vi "LSRS Drive.vi"(7 "Drive Side":enum16{"Right Side", "Left Side "}(ring), 10 "Inputs":dbl[](array[numeric])) -> (1 "Current Speed":dbl, 2 "Motor 2 Output":dbl, 3 "Motor Output":dbl)   [LabVIEW 2016]
uses:
  <vilib>/Rock Robotics/Network Tables/NT Read Number.vi
  <vilib>/Rock Robotics/Network Tables/NT Write Number.vi
  <vilib>/addons/control/pid/pid.llb/PID (DBL).vi
  <vilib>/addons/control/pid/NI_PID_pid.lvlib
panel:
  out "PID Values":cluster{"P":dbl, "I":dbl, "D":dbl}
  out "Right Button":bool
  out "Left Button":bool
  # "Left/Right Side Drive \nFRC Team 6364"
  # "Red is left side on."
  # "Blue is right side on."
  # "Adapted from Team 34`s Program"
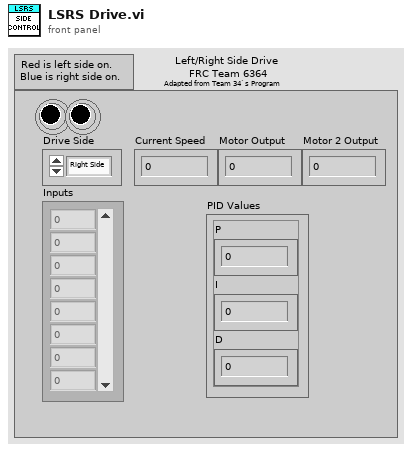
[diagram p1: front panel]
types:
  T1 = enum16{"Z", "Y", "X", "Rot. Point X", "Rot. Point Y", "Width/2", "Max", "Length/2"}
  T2 = typedef "WPI_EncoderDevRef.ctl" = cluster{"DevStatus":errorcluster, "EncoderIndex":T3, "CounterIndex":T4, "DistancePerCount":dbl, "Decoding Type":T5}
  T3 = typedef "FPGA_EncoderIdx.ctl" = enum8{"Enc 0", "Enc 1", "Enc 2", "Enc 3", "Enc 4", "Enc 5", "Enc 6", "Enc 7", "Invalid"}
  T4 = typedef "FPGA_CounterCtrSystemIndex.ctl" = enum8{"Ctr 0", "Ctr 1", "Ctr 2", "Ctr 3", "Ctr 4", "Ctr 5", "Ctr 6", "Ctr 7", "Invalid"}
  T5 = typedef "WPI_EncoderType.ctl" = enum16{"1x", "2x", "4x"}
  T6 = typedef "WPI_MotorControlDeviceRef.ctl" = cluster{"DeviceStatus":errorcluster, "Type":T7, "PWM":cluster{"PWM Channel":T8, "DeadBand":T9}, "CAN":cluster{"Device Number":u8, "SetOutput VI Ref":variant, "GetOutput VI Ref":variant, "Enable VI Ref":variant, "Disable VI Ref":variant, "Data":variant}, "Invert":bool}
  T7 = typedef "WPI_MotorControlType.ctl" = enum16{"PWM", "CAN"}
  T8 = typedef "FPGA_DIOPWMChannel.ctl" = enum8{"PWM 0", "PWM 1", "PWM 2", "PWM 3", "PWM 4", "PWM 5", "PWM 6", "PWM 7", "PWM 8", "PWM 9", "PWM MXP 0", "PWM MXP 1", "PWM MXP 2", "PWM MXP 3", "PWM MXP 4", "PWM MXP 5", "PWM MXP 6", "PWM MXP 7", "PWM MXP 8", "PWM MXP 9", "Invalid"}
  T9 = typedef "WPI_PWMDeadband.ctl" = cluster{"Name":string, "maxPositivePwm":i32, "minPositivePwm":i32, "centerPwm":i32, "maxNegativePwm":i32, "minNegativePwm":i32, "angularRange":u16}
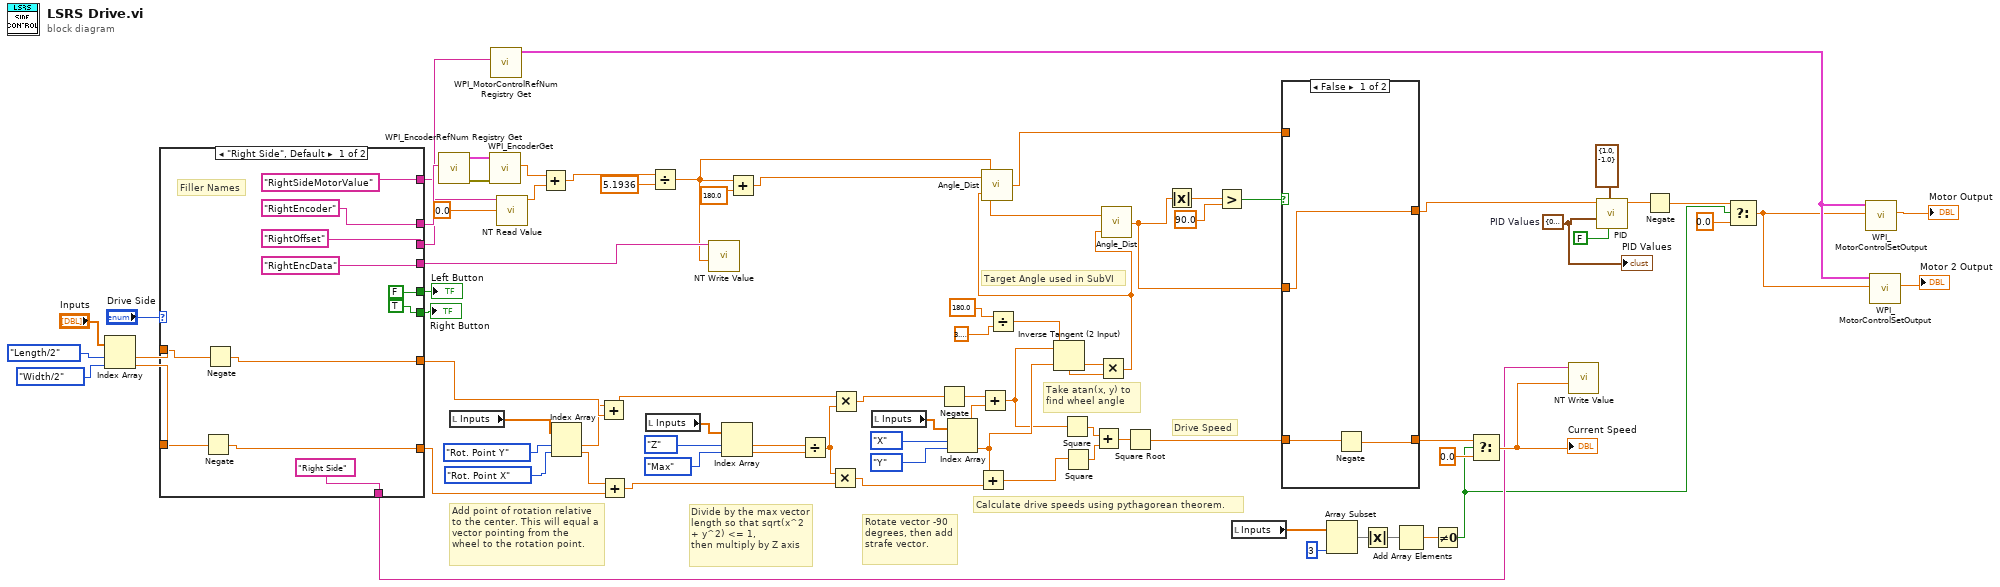
[diagram p0: block diagram]
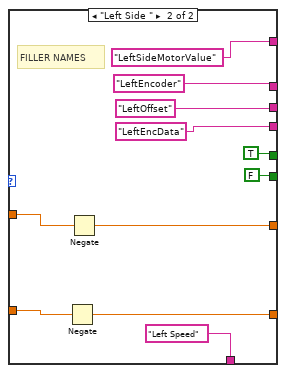
[diagram p3: hidden frame]
diagram:
  w3 = cluster{"P":dbl, "I":dbl, "D":dbl} {"P"=0.1, "I"=0.0, "D"=0.0}  # PID Values
  # "Drive Speed"
  # "Target Angle used in SubVI"
  # "Take atan(x, y) to find wheel angle"
  # "Rotate vector -90 degrees, then add strafe vector."
  # "Divide by the max vector length so that sqrt(x^2 + y^2) <= 1,\nthen multiply by Z axis"
  # "Add point of rotation relative to the center. This will equal a vector pointing from the\nwheel to the rotation point."
  # "Calculate drive speeds using pythagorean theorem."
  n1 = Index Array(array="Inputs", index #1=T1."Length/2", index #2=T1."Width/2") -> (element #1=w79:dbl, element #2=w78:dbl)
  n2 = case shown="\"Right Side\", Default" "Drive Side" {
    tunnel: w79 -> [w93 w102]
    tunnel: w78 -> [w91 w100]
    tunnel: ["RightSideMotorValue" ("refnum name") "LeftSideMotorValue" ("refnum name")] -> w63
    tunnel: ["RightEncoder" ("refnum name") "LeftEncoder" ("refnum name")] -> w75
    tunnel: [w92 w101] -> w67
    tunnel: [w90 w99] -> w64
    tunnel: ["RightOffset" ("refnum name") "LeftOffset" ("refnum name")] -> w74
    tunnel: ["RightEncData" ("refnum name") "LeftEncData" ("refnum name")] -> w59
    tunnel: [FALSE TRUE] -> w57
    tunnel: [TRUE FALSE] -> w56
    tunnel: ["Right Side" ("Name") "Left Speed" ("Name")] -> w12
    frame "Right Side", Default {
      # "Filler Names"
      n3 = Negate(x=w91) -> (-x=w90:dbl)
      n4 = Negate(x=w93) -> (-x=w92:dbl)
    }
    frame "Left Side " {
      # "FILLER NAMES"
      n5 = Negate(x=w100) -> (-x=w99:dbl)
      n6 = Negate(x=w102) -> (-x=w101:dbl)
    }
  }
  "Left Button" <- w57
  "Right Button" <- w56
  n7 = call <vilib>:"WPI_EncoderRefNum Registry Get.vi"("refnum name"=w75) -> ("error out"=w77:errorcluster, "EncoderDevRef"=w76:T2)  [unwired: 9 in]
  n8 = local read "Inputs"() -> (w70:dbl[])
  n9 = call <vilib>:"WPI_EncoderGet.vi"("error in (no error)"=w77, "EncoderDevRef"=w76) -> ("Distance"=w71:dbl)  [unwired: 4 in, 5 out]
  n10 = call <vilib>:"WPI_MotorControlRefNum Registry Get.vi"("refnum name"=w63) -> ("MotorControlDevRef"=w62:T6)  [unwired: 9 in, 1 out]
  n11 = call-poly <vilib>:"NT Read Value.vi"("Default Value"=0.0, "Name"=w74) -> ("Numeric"=w72:dbl)  [unwired: 8 in, 1 out]
  n12 = Add(x=w71, y=w72) -> (x+y=w61:dbl)
  n13 = Index Array(array=w70, index #1=T1."Rot. Point Y", index #2=T1."Rot. Point X") -> (element #1=w66:dbl, element #2=w65:dbl)
  n14 = Add(x=w66, y=w67) -> (x+y=w42:dbl)
  n15 = Add(x=w65, y=w64) -> (x+y=w40:dbl)
  n16 = local read "Inputs"() -> (w47:dbl[])
  n17 = Divide(x=w61, y=5.1936) -> (x/y=w52:dbl)
  n18 = call-poly <vilib>:"NT Write Value.vi"("Numeric"=w52, "Name"=w59) -> ()  [unwired: 9 in, 1 out]
  n19 = Index Array(array=w47, index #1=T1."Z", index #2=T1."Max") -> (element #1=w43:dbl, element #2=w44:dbl)
  n20 = Add(x=w52, y=180.0 ("upper limit")) -> (x+y=w54:dbl)
  n21 = Divide(x=w43, y=w44) -> (x/y=w41:dbl)
  n22 = Multiply(x=w41, y=w40) -> (x*y=w34:dbl)
  n23 = Multiply(x=w42, y=w41) -> (x*y=w36:dbl)
  n24 = local read "Inputs"() -> (w37:dbl[])
  n25 = Negate(x=w36) -> (-x=w35:dbl)
  n26 = Index Array(array=w37, index #1=T1."X", index #2=T1."Y") -> (element #1=w33:dbl, element #2=w32:dbl)
  n27 = Add(x=w32, y=w34) -> (x+y=w26:dbl)
  n28 = Add(x=w35, y=w33) -> (x+y=w27:dbl)
  n29 = Divide(x=180.0, y=3.141592653589793) -> (x/y=w29:dbl)
  n30 = Inverse Tangent (2 Input)(1:w32, 2:w27) -> (0:w28:dbl)
  n31 = Square(x=w27) -> (x^2=w24:dbl)
  n32 = Square(x=w26) -> (x^2=w25:dbl)
  n33 = Add(x=w24, y=w25) -> (x+y=w23:dbl)
  n34 = Multiply(x=w29, y=w28) -> (x*y=w22:dbl)
  n35 = call "Angle_Dist.vi"("TargetAngle"=w22, "CurrentAngle"=w54) -> ("Distance"=w53:dbl)
  n36 = call "Angle_Dist.vi"("TargetAngle"=w22, "CurrentAngle"=w52) -> ("Distance"=w48:dbl)
  n37 = Square Root(x=w23) -> (sqrt(x)=w21:dbl)
  n38 = Absolute Value(x=w48) -> (abs(x)=w51:dbl)
  n39 = Greater?(x=w51, y=90.0) -> (0:w49:bool)
  n40 = local read "Inputs"() -> (w19:dbl[])
  n41 = case shown="False" w49 {
    tunnel: w53 -> [_ w108]
    tunnel: w48 -> [w105 _]
    tunnel: w21 -> [w107 w109]
    tunnel: [w106 w109] -> w15
    tunnel: [w105 w108] -> w11
    frame False {
      n42 = Negate(x=w107) -> (-x=w106:dbl)
    }
    frame True {
    }
  }
  n43 = Array Subset(array=w19, length=3) -> (w17:dbl[])  [unwired: 1 in]
  n44 = Absolute Value(x=w17) -> (abs(x)=w18:dbl[])
  n45 = Add Array Elements(numeric array=w18) -> (sum=w16:dbl)
  n46 = Not Equal To 0?(x=w16) -> (x != 0?=w5:bool)
  n47 = Select(t=w15, s=w5, f=0.0) -> (s? t:f=w13:dbl)
  "Current Speed" <- w13
  n48 = call-poly <vilib>:"NT Write Value.vi"("Numeric"=w13, "Name"=w12) -> ()  [unwired: 9 in, 1 out]
  n49 = call-poly <vilib>:"PID.vi"("reinitialize? (F)"=FALSE, "output range"=cluster{"output high":dbl, "output low":dbl} {"output high"=1.0, "output low"=-1.0}, "PID gains"=w3, "setpoint"=w11) -> ("output"=w8:dbl)  [unwired: 6 in, 1 out]
  n50 = Negate(x=w8) -> (-x=w7:dbl)
  n51 = Select(t=w7, s=w5, f=0.0) -> (s? t:f=w4:dbl)
  n52 = call <vilib>:"WPI_MotorControlSetOutput.vi"("Output"=w4, "MotorControlDevRef"=w62) -> ("Motor Output"=→"Motor Output":dbl)  [unwired: 7 in, 2 out]
  n53 = call <vilib>:"WPI_MotorControlSetOutput.vi"("Output"=w4, "MotorControlDevRef"=w62) -> ("Motor Output"=→"Motor 2 Output":dbl)  [unwired: 7 in, 2 out]
  "PID Values" <- w3
